vi "Oriilas.vi"() -> ()   [LabVIEW 2017]
uses:
  <vilib>/Analysis/baseanly.llb/Mean (DBL).vi
  <vilib>/Analysis/NI_AALBase.lvlib
panel:
  out "appended array 2":dbl[](array[numeric])
  out "Array":i32[][](array[numeric])
  out "new picture 2":picture
  out "appended array":u32[][](array[numeric])
  out "new picture":picture
  out "output array":u32[](array[numeric])
  out "element":dbl
  out "Waveform Chart":cluster{"number: 0 to 1":dbl, "mean":dbl}(graph)
  in  "stop":bool
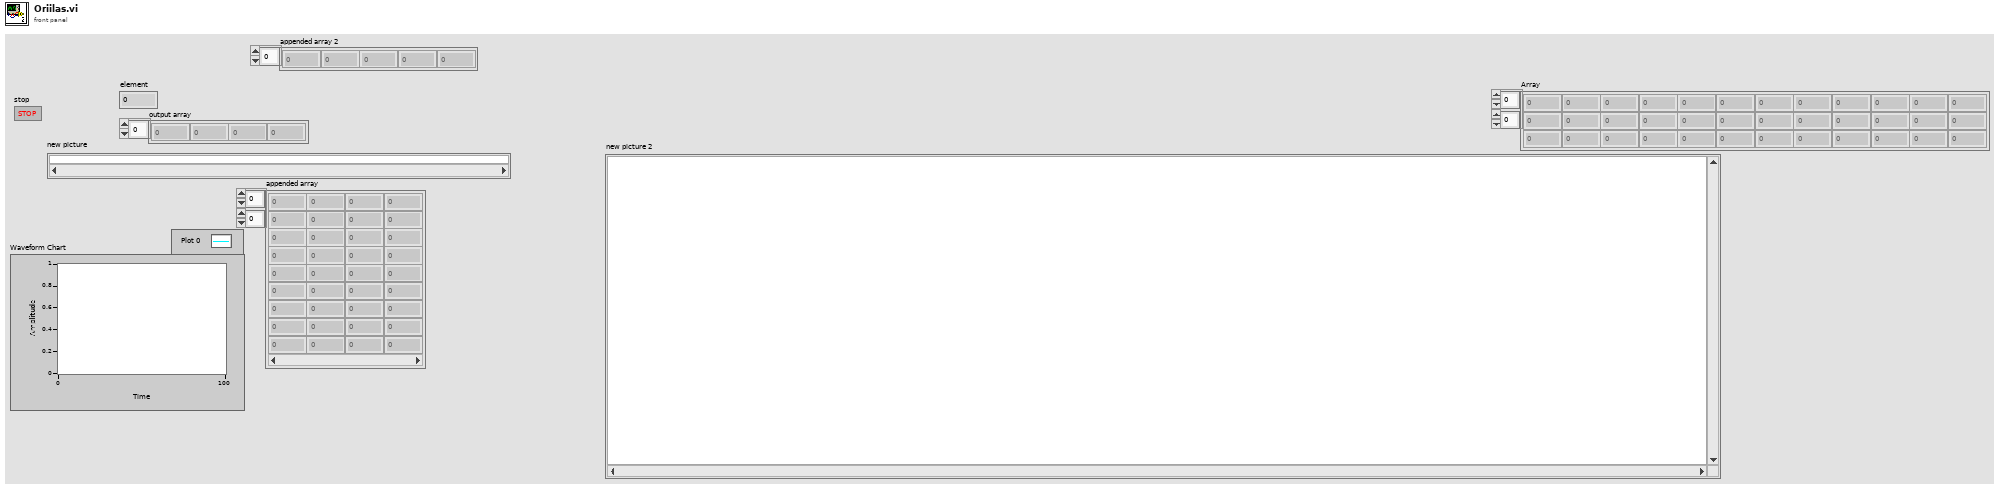
[diagram p1: front panel]
types:
  T1 = typedef "imagedata.ctl" = cluster{"image type":i32, "image depth":i32, "image":u8[], "mask":u8[], "colors":u32[], "Rectangle":cluster{"left":i16, "top":i16, "right":i16, "bottom":i16}}
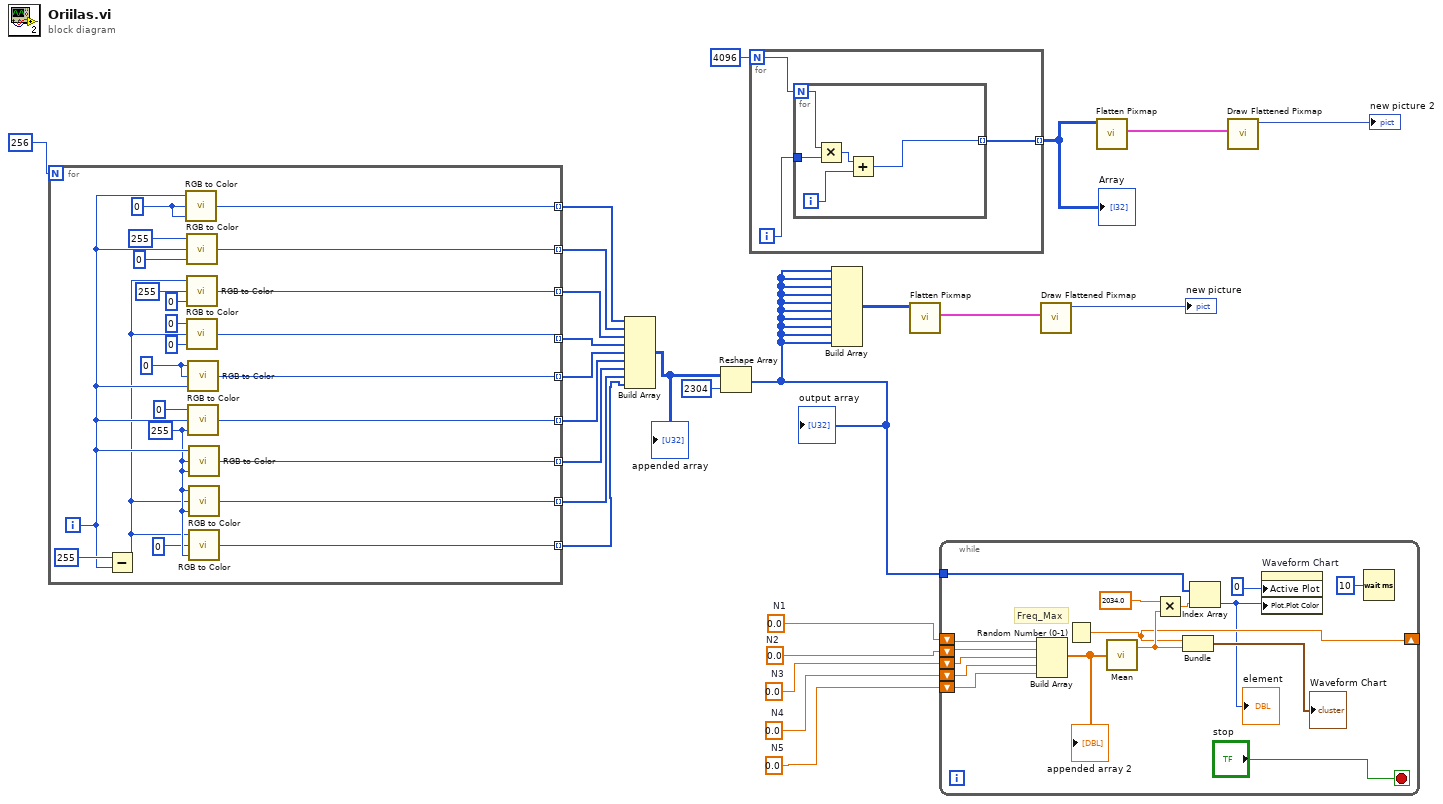
[diagram p0: block diagram]
diagram:
  w13 = 0.0  # N5
  w14 = 0.0  # N4
  w15 = 0.0  # N3
  w16 = 0.0  # N2
  w17 = 0.0  # N1
  n1 = for {
    N: 256 -> [_]
    tunnel: [w48] -> w6 mode=indexing
    tunnel: [w47] -> w5 mode=indexing
    tunnel: [w46] -> w24 mode=indexing
    tunnel: [w45] -> w23 mode=indexing
    tunnel: [w44] -> w22 mode=indexing
    tunnel: [w43] -> w21 mode=indexing
    tunnel: [w42] -> w20 mode=indexing
    tunnel: [w41] -> w19 mode=indexing
    tunnel: [w40] -> w18 mode=indexing
    i -> [w29]
    w28 = u8 255 ("B")
    w32 = u8 0 ("R")
    w31 = u8 0 ("G")
    n2 = Subtract(x=255, y=w29) -> (x-y=w26:i32)
    n3 = call <vilib>:"RGB to Color.vi"("B"=w31, "G"=w31, "R"=w29) -> ("Color"=w48:u32)
    n4 = call <vilib>:"RGB to Color.vi"("B"=u8 0, "G"=w29, "R"=u8 255) -> ("Color"=w47:u32)
    n5 = call <vilib>:"RGB to Color.vi"("B"=u8 0, "G"=u8 255, "R"=w26) -> ("Color"=w46:u32)
    n6 = call <vilib>:"RGB to Color.vi"("B"=u8 0, "G"=w26, "R"=u8 0) -> ("Color"=w45:u32)
    n7 = call <vilib>:"RGB to Color.vi"("B"=w29, "G"=w32, "R"=w32) -> ("Color"=w44:u32)
    n8 = call <vilib>:"RGB to Color.vi"("B"=w28, "G"=w29, "R"=u8 0 ("G")) -> ("Color"=w43:u32)
    n9 = call <vilib>:"RGB to Color.vi"("B"=w28, "G"=w28, "R"=w29) -> ("Color"=w42:u32)
    n10 = call <vilib>:"RGB to Color.vi"("B"=w28, "G"=w26, "R"=w28) -> ("Color"=w41:u32)
    n11 = call <vilib>:"RGB to Color.vi"("B"=w28, "G"=u8 0 ("R"), "R"=w26) -> ("Color"=w40:u32)
  }
  n12 = Build Array "Build Array"(w6, w5, w24, w23, w22, w21, w20, w19, w18) -> (w12:u32[][])
  "appended array" <- w12
  n13 = Reshape Array(w12, 2304 ("dimension size")) -> (w8:u32[])
  "output array" <- w8
  n14 = for {
    N: 4096 -> [w51]
    tunnel: [w49] -> w1 mode=indexing
    i -> [w50]
    n15 = for {
      N: w51 -> [w54]
      tunnel: w50 -> [w53]
      tunnel: [w52] -> w49 mode=indexing
      i -> [w56]
      n16 = Multiply(x=w54, y=w53) -> (x*y=w55:i32)
      n17 = Add(x=w55, y=w56) -> (x+y=w52:i32)
    }
  }
  "Array" <- w1
  n18 = Build Array(w8, w8, w8, w8, w8, w8, w8, w8, w8, w8) -> (w7:u32[][])
  n19 = call <vilib>:"Flatten Pixmap.vi"("24-bit pixmap"=w7) -> ("image data"=w10:T1)  [unwired: 10 in]
  n20 = while {
    shift-right: [w59] -> _
    shift-left: w17 -> [w71]
    shift-left: w16 -> [w70]
    shift-left: w15 -> [w69]
    shift-left: w14 -> [w68]
    shift-left: w13 -> [w67]
    tunnel: w8 -> [w58]
    stop <- "stop" stop-if-true
    # "Freq_Max"
    n21 = Build Array(w71, w70, w69, w68, w67) -> (w66:dbl[])
    "appended array 2" <- w66
    n22 = Random Number (0-1)() -> (number: 0 to 1=w59:dbl)
    n23 = call-poly <vilib>:"Mean.vi"("X"=w66) -> ("mean"=w60:dbl)  [unwired: 1 out]
    n24 = Multiply(x=2034.0, y=w60) -> (x*y=w64:dbl)
    n25 = Bundle("number: 0 to 1"=w59, "mean"=w60) -> (→"Waveform Chart":cluster{"number: 0 to 1":dbl, "mean":dbl})  [unwired: 1 in]
    n26 = Index Array(array=w58, index=w64) -> (element=w57:u32)
    "element" <- w57
    n27 = property on="Waveform Chart" class="WFChart (strict)"("Active Plot"=0, "Plot.Plot Color"=w57) -> ()  [unwired: 2 in, 2 out]
    n28 = Wait (ms)(milliseconds to wait=u32 10) -> ()  [unwired: 1 out]
  }
  n29 = call <vilib>:"Draw Flattened Pixmap.vi"("image data"=w10) -> ("new picture"=→"new picture":picture)  [unwired: 8 in]
  n30 = call <vilib>:"Flatten Pixmap.vi"("24-bit pixmap"=w1) -> ("image data"=w3:T1)  [unwired: 10 in]
  n31 = call <vilib>:"Draw Flattened Pixmap.vi"("image data"=w3) -> ("new picture"=→"new picture 2":picture)  [unwired: 8 in]
